vi "Create All Message Queues (Scale).vi"(8 "error in (no error)":errorcluster, 11 "Process Name":string) -> (0 "error out":errorcluster, 3 "Message Queues":T1)   [LabVIEW 2018, in "Sonicator Module.lvlib"]
uses:
  Sonicator Module.lvlib
  Sonicator Message Queues.ctl
  support/Message Queue/Message Cluster.ctl
  Feed Module/Controls/Sonicator Module Display.ctl
  support/Message Queue/Enqueue Message (Single).vi
  support/Message Queue/Message Queue.lvlib
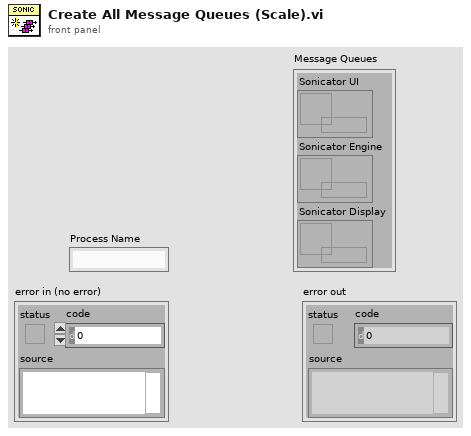
[diagram p1: front panel]
types:
  T1 = typedef "Sonicator Module.lvlib/Sonicator Message Queues.ctl" = cluster{"Sonicator UI":refnum<queue>, "Sonicator Engine":refnum<queue>, "Sonicator Display":refnum<queue>}
  T2 = typedef "Sonicator Module.lvlib/Sonicator Module Display.ctl" = cluster{"Pump On?":enum16{"Off", "On", "Not Initialized"}, "Sonicator Amp Value":dbl, "Sonicator Power Value":dbl, "Cycle Period":dbl}
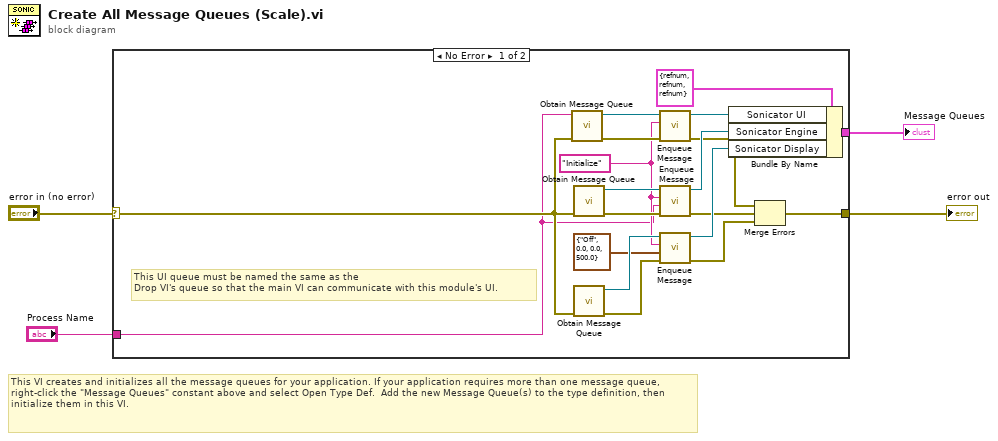
[diagram p0: block diagram]
diagram:
  # "This VI creates and initializes all the message queues for your application. If your application requires more than one message queue, right-click the \"Message Queues\" constant above and select Open Type Def.  Add the new Message Queue(s) to the type definition, then initialize them in this VI."
  n1 = case shown="No Error" "error in (no error)" {
    selector: "error in (no error)" -> [w8 w24]
    tunnel: [w22 w24] -> w4
    tunnel: [w23 _] -> w3
    tunnel: "Process Name" -> [w5 _]
    frame No Error {
      w6 = "Initialize" ("Message")
      # "This UI queue must be named the same as the \nDrop VI's queue so that the main VI can communicate with this module's UI."
      n2 = call "Obtain Message Queue.vi"("error in (no error)"=w8, "name (unnamed)"=w5) -> ("error out"=w18:errorcluster, "Message Queue"=w21:refnum<queue>)  [unwired: 8 in]
      n3 = call "Obtain Message Queue.vi"("error in (no error)"=w8) -> ("error out"=w17:errorcluster, "Message Queue"=w20:refnum<queue>)  [unwired: 9 in]
      n4 = call "Obtain Message Queue.vi"("error in (no error)"=w8) -> ("error out"=w16:errorcluster, "Message Queue"=w19:refnum<queue>)  [unwired: 9 in]
      n5 = call-poly "Enqueue Message.vi"("error in (no error)"=w18, "Message"=w6, "Message Queue"=w21) -> ("error out"=w12:errorcluster, "dup Message Queue"=w15:refnum<queue>)  [unwired: 7 in]
      n6 = call-poly "Enqueue Message.vi"("error in (no error)"=w17, "Message Data"=w5, "Message"=w6, "Message Queue"=w20) -> ("error out"=w11:errorcluster, "dup Message Queue"=w14:refnum<queue>)  [unwired: 6 in]
      n7 = call-poly "Enqueue Message.vi"("error in (no error)"=w16, "Message Data"=T2 {"Pump On?"=enum."Off", "Sonicator Amp Value"=0.0, "Sonicator Power Value"=0.0, "Cycle Period"=500.0} ("SM Display"), "Message"=w6, "Message Queue"=w19) -> ("error out"=w10:errorcluster, "dup Message Queue"=w13:refnum<queue>)  [unwired: 6 in]
      n8 = Bundle By Name(cluster=T1 {"Sonicator UI"=refnum, "Sonicator Engine"=refnum, "Sonicator Display"=refnum} ("Message Queues"), "Sonicator UI"=w15, "Sonicator Engine"=w14, "Sonicator Display"=w13) -> (w23:T1)
      n9 = Merge Errors(w12, w11, w10) -> (w22:errorcluster)
    }
    frame Error {
    }
  }
  "Message Queues" <- w3
  "error out" <- w4
